vi "Execute Callback.vi"(8 "Write Status":errorcluster, 11 "IWriteExecutionPolicy in":refnum<class "Synchronous Write Callback.lvclass">) -> ()   [LabVIEW 2020, in "Network Messenger.lvlib" / "Synchronous Write Callback.lvclass"]
uses:
  <vilib>/gpm_packages/@cs/Network-interface/Source/Network Messenger/Synchronous Write Callback/Synchronous Write Callback.lvclass
  <vilib>/gpm_packages/@cs/Network-interface/Source/Network Messenger/Synchronous Write Callback/Synchronous Write Callback.lvclass/Synchronous Write Callback.ctl
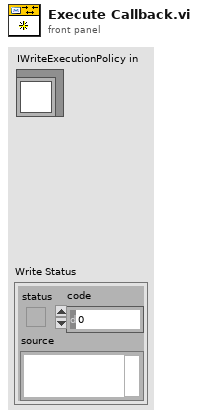
[diagram p1: front panel]
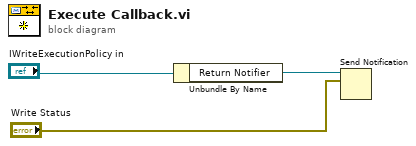
[diagram p0: block diagram]
diagram:
  n1 = Unbundle By Name("IWriteExecutionPolicy in") -> ("Return Notifier"=w2:refnum<notifier>)
  n2 = Send Notification(notification="Write Status", notifier=w2) -> ()  [unwired: 1 in, 2 out]
